vi "LaserGetPower.vi"(7 "error in (no error)":errorcluster, 10 "reference In":refnum<k24>) -> (0 "error out":errorcluster, 2 "Power":cluster{"Time":dbl, "Power":dbl}, 3 "reference out":refnum<k24>)   [LabVIEW 2019]
doc: "Generates sample waveforms according to the signal type in the HW Config input."
uses:
  E:/DevHardSoftware/MMicroscopy/HardwareAdapter/Lasers/Dependencies/Oxxius_Boxx.dll
  Dependencies/Oxxius_Boxx.dll
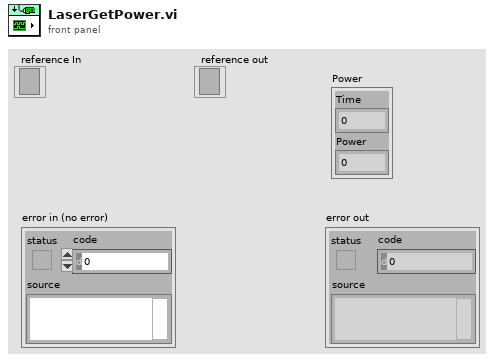
[diagram p1: front panel]
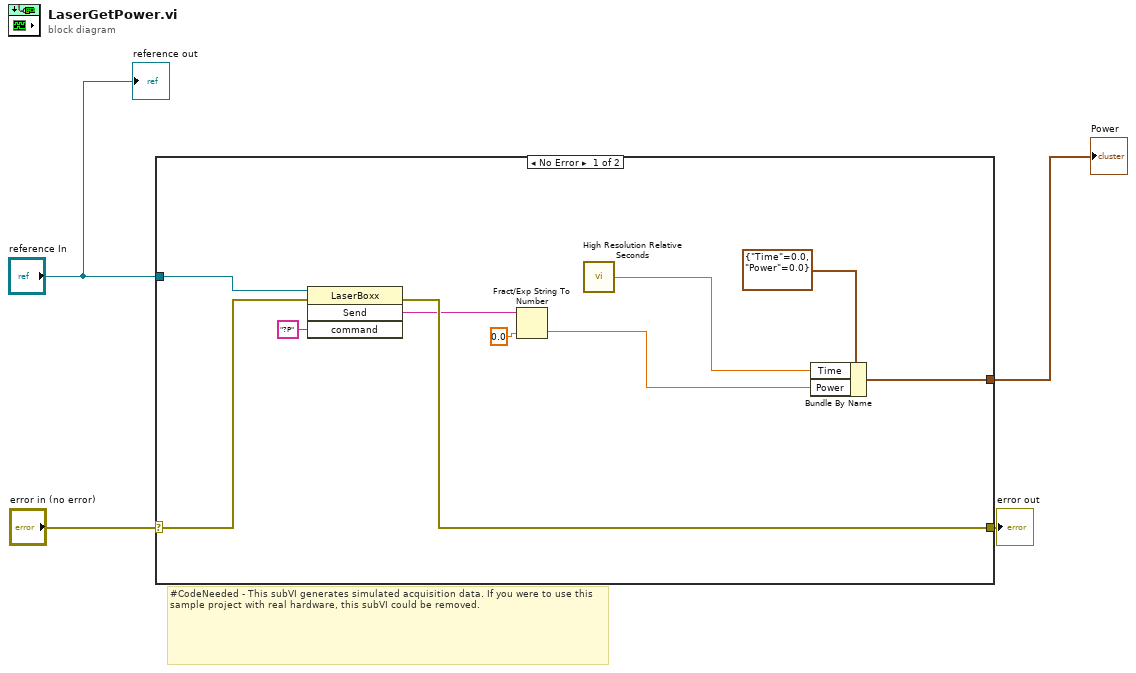
[diagram p0: block diagram]
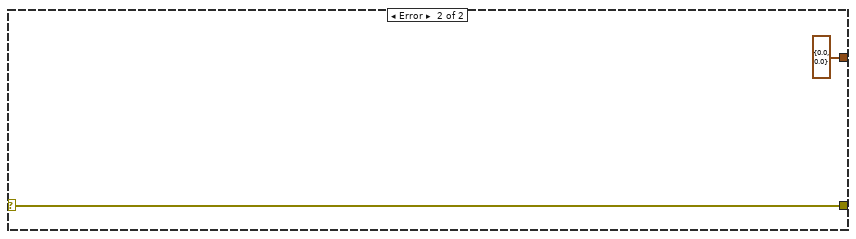
[diagram p2: hidden frame]
diagram:
  # "#CodeNeeded - This subVI generates simulated acquisition data. If you were to use this sample project with real hardware, this subVI could be removed."
  n1 = case shown="No Error" "error in (no error)" {
    selector: "error in (no error)" -> [w12 w16]
    tunnel: [w11 w16] -> w3
    tunnel: "reference In" -> [w13 _]
    tunnel: [w8 cluster{"Time":dbl, "Power":dbl} {"Time"=0.0, "Power"=0.0} ("RawImage")] -> w1
    frame No Error {
      n2 = invoke class="LaserBoxx" method="Send"(reference=w13, error in=w12, "command"="?P") -> (error out=w11:errorcluster, "Send"=w5:string)  [unwired: 1 in, 2 out]
      n3 = Fract/Exp String To Number(string=w5, default (0 dbl)=0.0 ("default (0 DBL)")) -> (number=w7:dbl)  [unwired: 2 in, 1 out]
      n4 = call <vilib>:"High Resolution Relative Seconds.vi"() -> ("relative seconds"=w10:dbl)
      n5 = Bundle By Name(cluster=cluster{"Time":dbl, "Power":dbl} {"Time"=0.0, "Power"=0.0} ("RawImage"), "Time"=w10, "Power"=w7) -> (w8:cluster{"Time":dbl, "Power":dbl})
    }
    frame Error {
    }
  }
  "error out" <- w3
  "Power" <- w1
  "reference out" <- "reference In"
